vi "sorted by gradient of fitted straight line.vi"(0 "cases CSV":string[][](array[string]), 5 "US data":T1, 7 "Populations":i32[](array[numeric]), 9 "deaths CSV":string[][](array[string]), 11 "filter out":i32[](array[numeric])) -> (4 "country index array for cases (gained)":i32[](array[numeric]), 6 "country index for deaths (gained)":i32[](array[numeric]), 8 "country index array for cases (dropped)":i32[](array[numeric]), 10 "country index for deaths (dropped)":i32[](array[numeric]))   [LabVIEW 2019]
uses:
  <vilib>/Analysis/NI_AALPro.lvlib
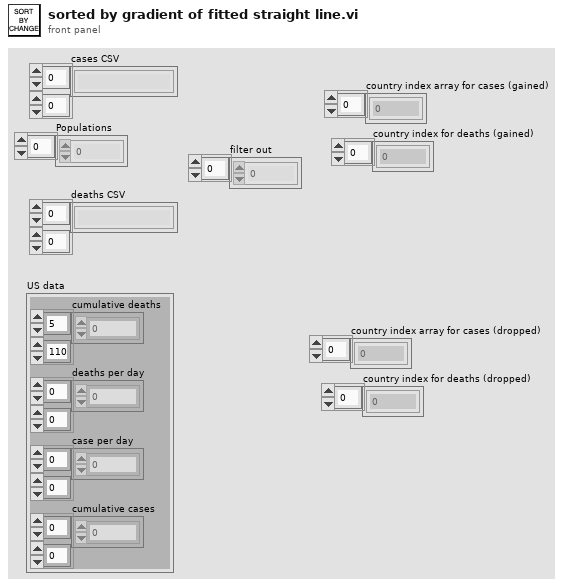
[diagram p1: front panel]
types:
  T1 = cluster{"cumulative deaths":i32[][], "deaths per day":i32[][], "case per day":i32[][], "cumulative cases":i32[][]}
  T2 = cluster{"percentage change":dbl, "country index":i32}
  T3 = cluster{"percentage change":dbl, "country index":i32}[]
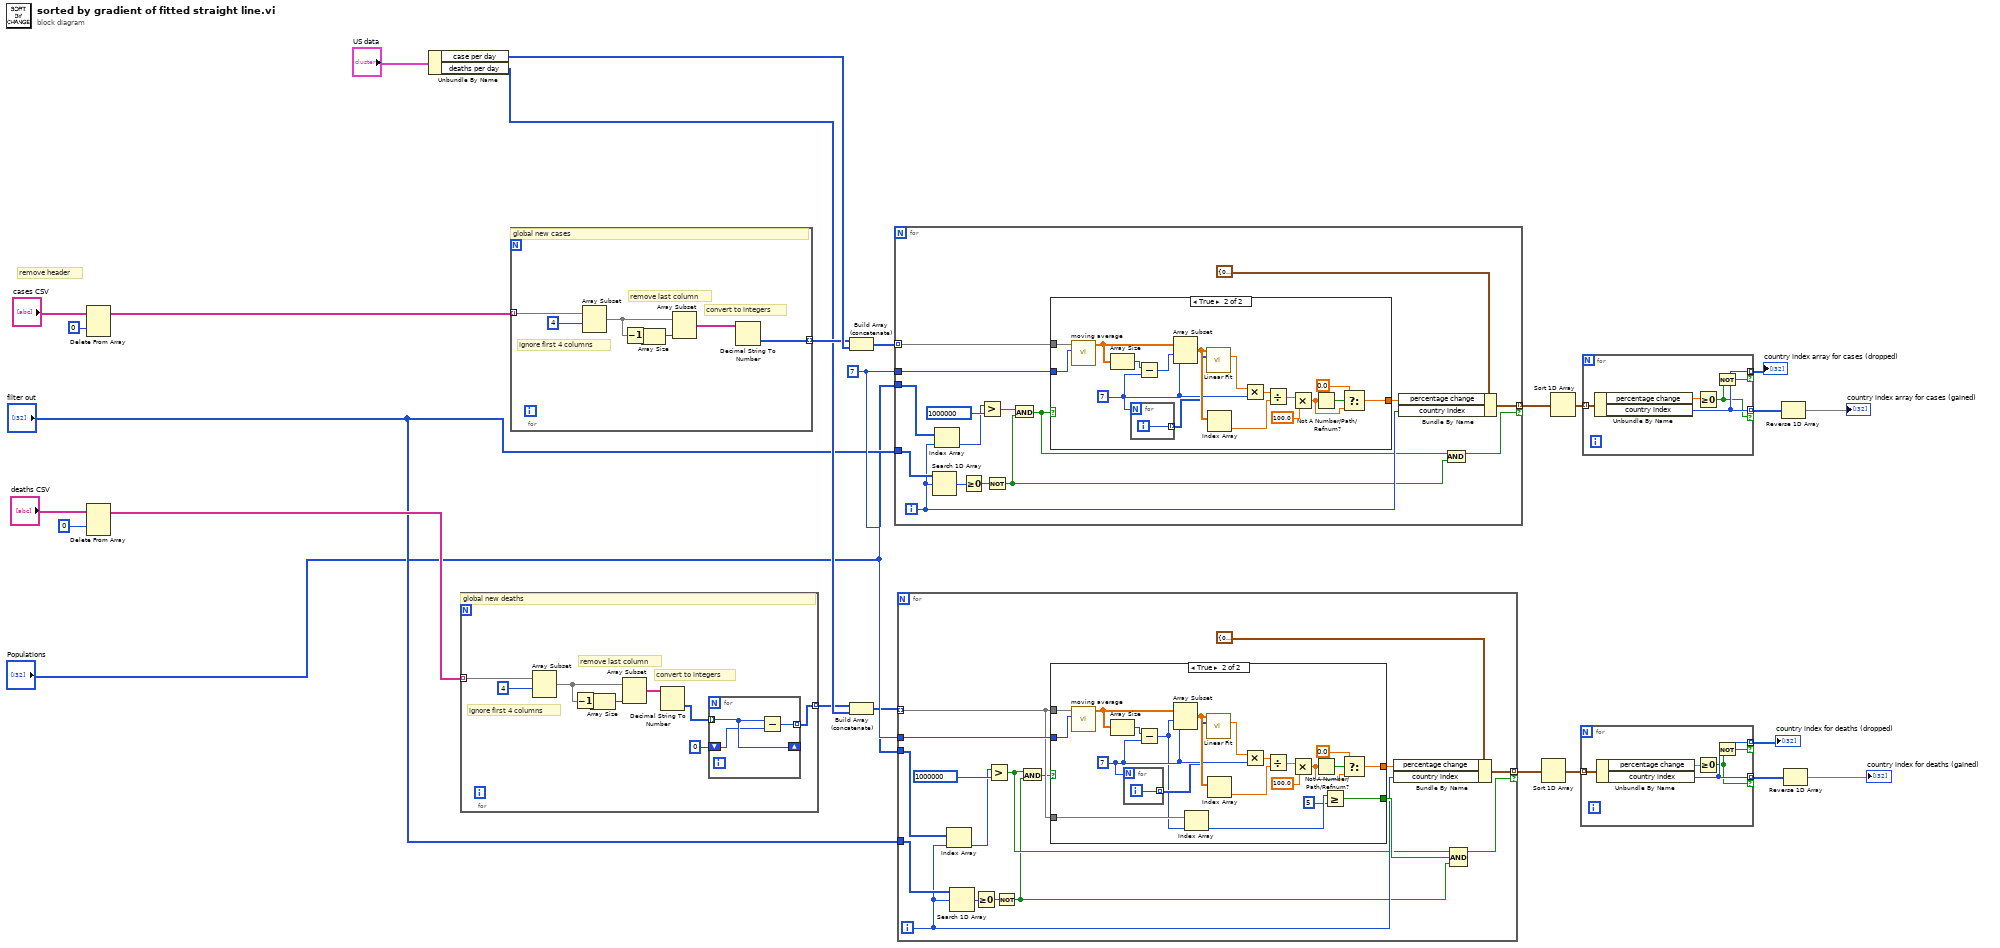
[diagram p0: block diagram]
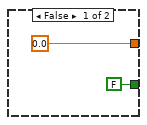
[diagram p2: hidden frame]
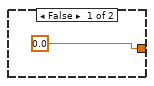
[diagram p3: hidden frame]
diagram:
  w13 = 7 ("average over x points")
  # "remove header"
  n1 = Delete From Array(array="cases CSV", index (row)=0) -> (array with subset deleted=w8:string[][])  [unwired: 2 in, 1 out]
  n2 = Delete From Array(array="deaths CSV", index (row)=0) -> (array with subset deleted=w7:string[][])  [unwired: 2 in, 1 out]
  n3 = Unbundle By Name("US data") -> ("case per day"=w21:i32[][], "deaths per day"=w15:i32[][])
  n4 = for {
    tunnel: w7 -> [w30] mode=indexing
    tunnel: [w27] -> w14 mode=indexing
    # "remove last column"
    # "convert to integers"
    # "ignore first 4 columns"
    # "global new deaths"
    n5 = Array Subset(array=w30, index=4) -> (w33:string[])  [unwired: 1 in]
    n6 = Array Size(array=w33) -> (size(s)=w31:i32)
    n7 = Decrement(x=w31) -> (x-1=w32:i32)
    n8 = Array Subset(array=w33, length=w32) -> (w34:string[])  [unwired: 1 in]
    n9 = Decimal String To Number(string=w34) -> (number=w28:i32[])  [unwired: 2 in, 1 out]
    n10 = for {
      tunnel: w28 -> [w38] mode=indexing
      shift-right: [w38] -> _
      shift-left: 0 -> [w37]
      tunnel: [w36] -> w27 mode=indexing
      n11 = Subtract(x=w38, y=w37) -> (x-y=w36:i32)
    }
  }
  n12 = for {
    tunnel: w8 -> [w40] mode=indexing
    tunnel: [w39] -> w20 mode=indexing
    # "remove last column"
    # "convert to integers"
    # "ignore first 4 columns"
    # "global new cases"
    n13 = Array Subset(array=w40, index=4) -> (w43:string[])  [unwired: 1 in]
    n14 = Array Size(array=w43) -> (size(s)=w41:i32)
    n15 = Decrement(x=w41) -> (x-1=w42:i32)
    n16 = Array Subset(array=w43, length=w42) -> (w44:string[])  [unwired: 1 in]
    n17 = Decimal String To Number(string=w44) -> (number=w39:i32[])  [unwired: 2 in, 1 out]
  }
  n18 = Build Array (concatenate)(w20, w21) -> (w19:i32[][])
  n19 = Build Array (concatenate)(w14, w15) -> (w10:i32[][])
  n20 = for {
    tunnel: w19 -> [w61] mode=indexing
    tunnel: w13 -> [w60]
    tunnel: "Populations" -> [w51]
    tunnel: [w56] -> w18 mode=indexing if=w53
    tunnel: "filter out" -> [w55]
    i -> [w49]
    n21 = Search 1D Array(1D array=w55, element=w49) -> (index of element=w54:i32)  [unwired: 1 in]
    n22 = Index Array(array=w51, index=w49) -> (element=w50:i32)
    n23 = Greater Or Equal To 0?(x=w54) -> (x >= 0?=w52:bool)
    n24 = Greater?(x=w50, y=1000000) -> (0:w48:bool)
    n25 = Not(x=w52) -> (.not. x?=w46:bool)
    n26 = And(x=w48, y=w46) -> (x .and. y?=w47:bool)
    n27 = case shown="True" w47 {
      tunnel: w61 -> [_ w79]
      tunnel: w60 -> [_ w78]
      tunnel: [0.0 w63] -> w57
      frame False {
      }
      frame True {
        w68 = 7 ("y")
        n28 = call "moving average.vi"("average over x points"=w78, "Array"=w79) -> ("moving average array"=w77:dbl[])  [unwired: 8 in, 1 out]
        n29 = Array Size(array=w77) -> (size(s)=w76:i32)
        n30 = for {
          N: w68 -> [_]
          tunnel: [w80] -> w67 mode=indexing
          i -> [w80]
        }
        n31 = Subtract(x=w76, y=w68) -> (x-y=w75:i32)
        n32 = Array Subset(array=w77, index=w75, length=w68) -> (w72:dbl[])
        n33 = call <vilib>:"Linear Fit.vi"("Y"=w72, "X"=w67) -> ("slope"=w74:dbl)  [unwired: 9 in, 4 out]
        n34 = Index Array(array=w72) -> (element=w71:dbl)  [unwired: 1 in]
        n35 = Multiply(x=w74, y=w68) -> (x*y=w73:dbl)
        n36 = Divide(x=w73, y=w71) -> (x/y=w70:dbl)
        n37 = Multiply(x=w70, y=100.0) -> (x*y=w64:dbl)
        n38 = Not A Number/Path/Refnum?(number/path/refnum=w64) -> (NaN/Path/Refnum?=w65:bool)
        n39 = Select(t=0.0, s=w65, f=w64) -> (s? t:f=w63:dbl)
      }
    }
    n40 = Bundle By Name(cluster=T2 {"percentage change"=0.0, "country index"=0}, "percentage change"=w57, "country index"=w49) -> (w56:T2)
    n41 = And(x=w47, y=w46) -> (x .and. y?=w53:bool)
  }
  n42 = for {
    tunnel: w10 -> [w91] mode=indexing
    tunnel: w13 -> [w97]
    tunnel: "Populations" -> [w85]
    tunnel: [w93] -> w11 mode=indexing if=w92
    tunnel: "filter out" -> [w87]
    i -> [w86]
    n43 = Index Array(array=w85, index=w86) -> (element=w84:i32)
    n44 = Search 1D Array(1D array=w87, element=w86) -> (index of element=w88:i32)  [unwired: 1 in]
    n45 = Greater Or Equal To 0?(x=w88) -> (x >= 0?=w89:bool)
    n46 = Greater?(x=w84, y=1000000) -> (0:w82:bool)
    n47 = Not(x=w89) -> (.not. x?=w81:bool)
    n48 = And(x=w82, y=w81) -> (x .and. y?=w83:bool)
    n49 = case shown="True" w83 {
      tunnel: w91 -> [_ w120]
      tunnel: w97 -> [_ w119]
      tunnel: [0.0 w108] -> w94
      tunnel: [FALSE w105] -> w90
      tunnel: w91 -> [_ w104]
      frame False {
      }
      frame True {
        w113 = 7 ("y")
        n50 = call "moving average.vi"("average over x points"=w119, "Array"=w120) -> ("moving average array"=w118:dbl[])  [unwired: 8 in, 1 out]
        n51 = Array Size(array=w118) -> (size(s)=w117:i32)
        n52 = for {
          N: w113 -> [_]
          tunnel: [w121] -> w112 mode=indexing
          i -> [w121]
        }
        n53 = Subtract(x=w117, y=w113) -> (x-y=w103:i32)
        n54 = Array Subset(array=w118, index=w103, length=w113) -> (w115:dbl[])
        n55 = Index Array(array=w104, index=w103) -> (element=w102:i32)
        n56 = call <vilib>:"Linear Fit.vi"("Y"=w115, "X"=w112) -> ("slope"=w101:dbl)  [unwired: 9 in, 4 out]
        n57 = Index Array(array=w115) -> (element=w107:dbl)  [unwired: 1 in]
        n58 = Multiply(x=w101, y=w113) -> (x*y=w116:dbl)
        n59 = Divide(x=w116, y=w107) -> (x/y=w114:dbl)
        n60 = Multiply(x=w114, y=100.0) -> (x*y=w109:dbl)
        n61 = Not A Number/Path/Refnum?(number/path/refnum=w109) -> (NaN/Path/Refnum?=w111:bool)
        n62 = Greater Or Equal?(x=w102, y=5) -> (x >= y?=w105:bool)
        n63 = Select(t=0.0, s=w111, f=w109) -> (s? t:f=w108:dbl)
      }
    }
    n64 = Bundle By Name(cluster=T2 {"percentage change"=0.0, "country index"=0}, "percentage change"=w94, "country index"=w86) -> (w93:T2)
    n65 = Compound Arithmetic op=AND(w82, w90, w81) -> (w92:bool)
  }
  n66 = Sort 1D Array(array=w11) -> (sorted array=w9:T3)
  n67 = Sort 1D Array(array=w18) -> (sorted array=w17:T3)
  n68 = for {
    tunnel: w9 -> [w126] mode=indexing
    tunnel: [w125] -> w12 mode=indexing if=w122
    tunnel: [w125] -> w4 mode=indexing if=w124
    n69 = Unbundle By Name(w126) -> ("percentage change"=w123:dbl, "country index"=w125:i32)
    n70 = Greater Or Equal To 0?(x=w123) -> (x >= 0?=w122:bool)
    n71 = Not(x=w122) -> (.not. x?=w124:bool)
  }
  "country index for deaths (dropped)" <- w4
  n72 = for {
    tunnel: w17 -> [w131] mode=indexing
    tunnel: [w129] -> w16 mode=indexing if=w127
    tunnel: [w129] -> w5 mode=indexing if=w128
    n73 = Unbundle By Name(w131) -> ("percentage change"=w130:dbl, "country index"=w129:i32)
    n74 = Greater Or Equal To 0?(x=w130) -> (x >= 0?=w127:bool)
    n75 = Not(x=w127) -> (.not. x?=w128:bool)
  }
  "country index array for cases (dropped)" <- w5
  n76 = Reverse 1D Array(array=w16) -> (reversed array=→"country index array for cases (gained)":i32[])
  n77 = Reverse 1D Array(array=w12) -> (reversed array=→"country index for deaths (gained)":i32[])
